vi "Clear DAQmx Tasks.vi"(8 "error in (no error)":errorcluster) -> (0 "error out":errorcluster)   [LabVIEW 2020]
uses:
  Triggers/Globals/gl_Triggering globals.vi
panel:
  out "Array":errorcluster[](array[cluster])
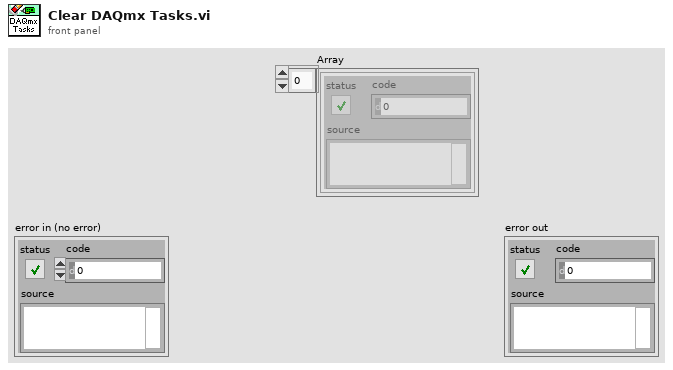
[diagram p1: front panel]
types:
  T1 = typedef "Triggered tasks cluster.ctl" = cluster{"DO task-Encoder trigger":refnum<k21>, "AO Task-Pockels modulation":refnum<k21>, "Counter Clock Task":refnum<k21>}
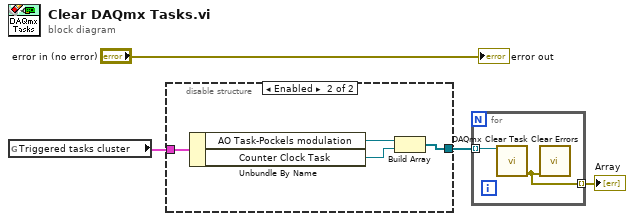
[diagram p0: block diagram]
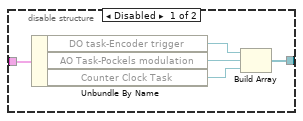
[diagram p2: hidden frame]
diagram:
  n1 = global read "gl_Triggering globals.vi" "Triggered tasks cluster"() -> (w3:T1)
  n2 = disable-structure shown="Enabled" {
    disable-tunnel: w3 -> [w9 w13]
    disable-tunnel: [w5 w10] -> w2
    frame Disabled {
      n3 = Unbundle By Name(w9) -> ("DO task-Encoder trigger"=w6:refnum<k21>, "AO Task-Pockels modulation"=w8:refnum<k21>, "Counter Clock Task"=w7:refnum<k21>)
      n4 = Build Array(w6, w8, w7) -> (w5:refnum<k21>[])
    }
    frame Enabled {
      n5 = Unbundle By Name(w13) -> ("AO Task-Pockels modulation"=w12:refnum<k21>, "Counter Clock Task"=w11:refnum<k21>)
      n6 = Build Array(w12, w11) -> (w10:refnum<k21>[])
    }
  }
  n7 = for {
    tunnel: w2 -> [w15] mode=indexing
    tunnel: [w14] -> w1 mode=indexing
    n8 = call <vilib>:"DAQmx Clear Task.vi"("task in"=w15) -> ("error out"=w14:errorcluster)  [unwired: 14 in]
    n9 = call <vilib>:"Clear Errors.vi"("error in (no error)"=w14) -> ()  [unwired: 5 in, 2 out]
  }
  "Array" <- w1
  "error out" <- "error in (no error)"
